vi "Wait for stop.vi"(1 "Port":T1={"P type"=0, "reference"="", " Terminator "="\r\n", "Timeout"=300} {"Timeout" step=10; "P type" items=["none", "RS-232C"]}, 3 "error in (no error)":errorcluster, 4 "wait for in pos":bool, 5 "Controller #":string) -> (9 "error out":errorcluster)   [LabVIEW 2021]
panel:
  out "In position?":bool
  out "Moving?":bool
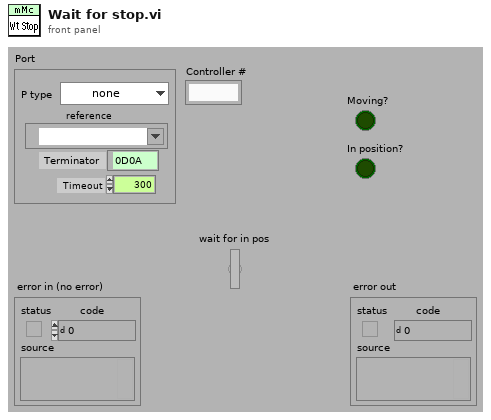
[diagram p1: front panel]
types:
  T1 = cluster{"P type":u16, "reference":refnum<visa-resource-name>, " Terminator ":string, "Timeout":i32}
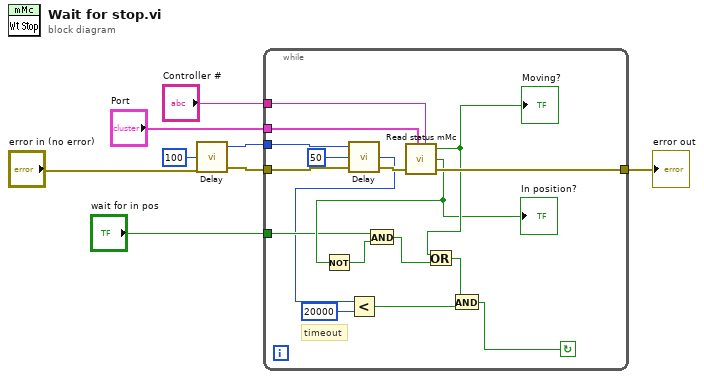
[diagram p0: block diagram]
diagram:
  n1 = call "Delay.vi"("milliseconds to wait"=u32 100, "error in (no error)"="error in (no error)") -> ("new time"=w1:u32, "error out"=w3:errorcluster)  [unwired: 5 in, 1 out]
  n2 = while {
    tunnel: "Port" -> [w25]
    tunnel: "Controller #" -> [w24]
    tunnel: [w23] -> w6
    tunnel: w3 -> [w22]
    tunnel: "wait for in pos" -> [w16]
    tunnel: w1 -> [w15]
    stop <- w9 continue-if-true
    # "timeout"
    n3 = call "Delay.vi"("old timer value"=w15, "milliseconds to wait"=u32 50, "error in (no error)"=w22) -> ("elapsed time"=w13:u32, "error out"=w21:errorcluster)  [unwired: 4 in, 1 out]
    n4 = Less?(x=w13, y=u32 20000) -> (x < y?=w11:bool)
    n5 = call "Read status mMc.vi"("Port"=w25, "error in (no error)"=w21, "Controller #"=w24) -> ("Moving?"=w19:bool, "In position?"=w18:bool, "error out"=w23:errorcluster)  [unwired: 4 in]
    "Moving?" <- w19
    "In position?" <- w18
    n6 = Not(x=w18) -> (.not. x?=w14:bool)
    n7 = And(x=w16, y=w14) -> (x .and. y?=w17:bool)
    n8 = Or(x=w19, y=w17) -> (x .or. y?=w10:bool)
    n9 = And(x=w10, y=w11) -> (x .and. y?=w9:bool)
  }
  "error out" <- w6
